vi "Interface Browser.vi"(5 "Caller VI Refnum (Callee's Caller)":refnum<vi>, 7 "Name(\"\" to use uuid)":string="interface_browser") -> ()   [LabVIEW 2017]
uses:
  _Support/Priority Queue/Priority Queue.lvclass/Priority Queue.ctl
  <vilib>/Utility/miscctls.llb/LVPointTypeDef.ctl
  AdvanceAPI/CSM - Check If Module Exists.vi
  Utility/Build Error Cluster.vi
  AdvanceAPI/CSM - Revert Arguments-Safe String.vi
  _Support/Common/Trim Single line Text.vi
  AdvanceAPI/CSM - Make String Arguments Safe.vi
  AdvanceAPI/CSM - Break Down Multiple States String.vi
  AdvanceAPI/CSM - Compact Multiple States.vi
  _Support/CSMQ/_Obtain CSM Data Queue.vi
  _Support/Priority Queue/Release Priority Queue.vi
  AdvanceAPI/CSM - Keywords.vi
  _Support/Priority Queue/Obtain Priority Queue.vi
  _csmHelper/API/Create From VI Reference.vi
  _csmHelper/API/Open Front Panel.vi
  _csmHelper/API/Destroy.vi
  _Support/Error/CSM No Target Error.vi
  _Polymophic/CSM - Filter Duplicated Lines.vi
  _Support/Priority Queue/Priority Queue.lvclass
  Communicable State Machine.lvlib
  _csmHelper/API with lvcsm Support/CSM-Helper API with lvcsm Support.lvlib
  _csmHelper/CSM-Helper.lvclass
  _csmHelper/lvcsmFile/lvcsm File Support.lvlib
panel:
  in  "Opton:All-CSM-VIs":bool
  in  "Scan Project":bool
  in  "Refresh":bool
  in  "Fast Forward":bool
  in  "Fast Reverse":bool
  in  "Skip to Beginning":bool
  in  "Skip to End":bool
  in  "Stop":bool
  in  "Play":bool
  in  "Open":bool
  in  "MainTree":string[](tree)
  in  "Interface-Filter":enum16{"API-Only", "UserDef States", "All"}(ring)=enum."UserDef States"
  in  "CSM-States":i32[](listbox)
  out "StateInfo@Image":string
  out "2D Picture":picture
  out "String":string
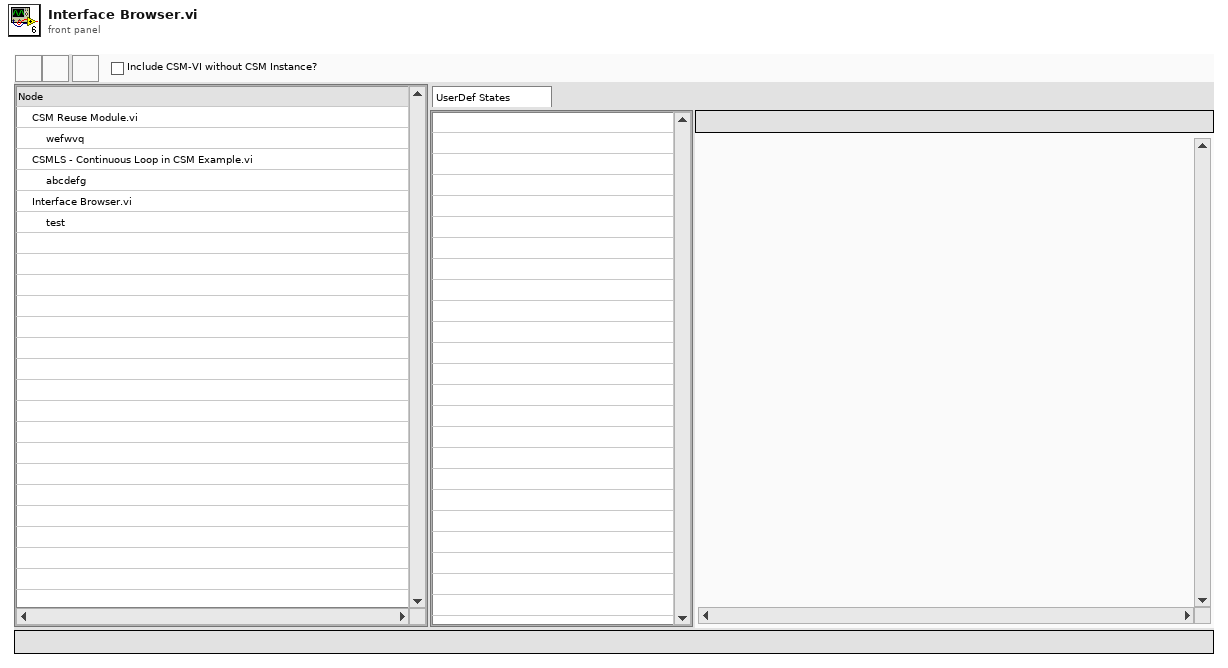
[diagram p1: front panel]
types:
  T1 = enum32{"Invalid", "Standard", "Closed", "Hidden", "Minimized", "Maximized"}
  T2 = enum32{"invalid app kind", "Development System", "Run Time System", "Student Edition", "Embedded LabVIEW", "Evaluation", "Custom"}
  T3 = typedef "LVPointTypeDef.ctl" = cluster{"Horizontal":i16, "Vertical":i16}
  T4 = typedef "Communicable State Machine.lvlib/_CSM_Response Source Message.ctl" = cluster{"‘State":string, "’Arguments":string, "’Error":errorcluster}
  T5 = cluster{"Current VI Reference":refnum<vi>, "Close Panel on Exit?":bool}
  T6 = cluster{"Core":cluster{"Current VI Reference":refnum<vi>, "Close Panel on Exit?":bool}, "Your Boolean data":bool, "Your string data":string}
  T7 = typedef "LVPoint32TypeDef.ctl" = cluster{"Horizontal":i32, "Vertical":i32}
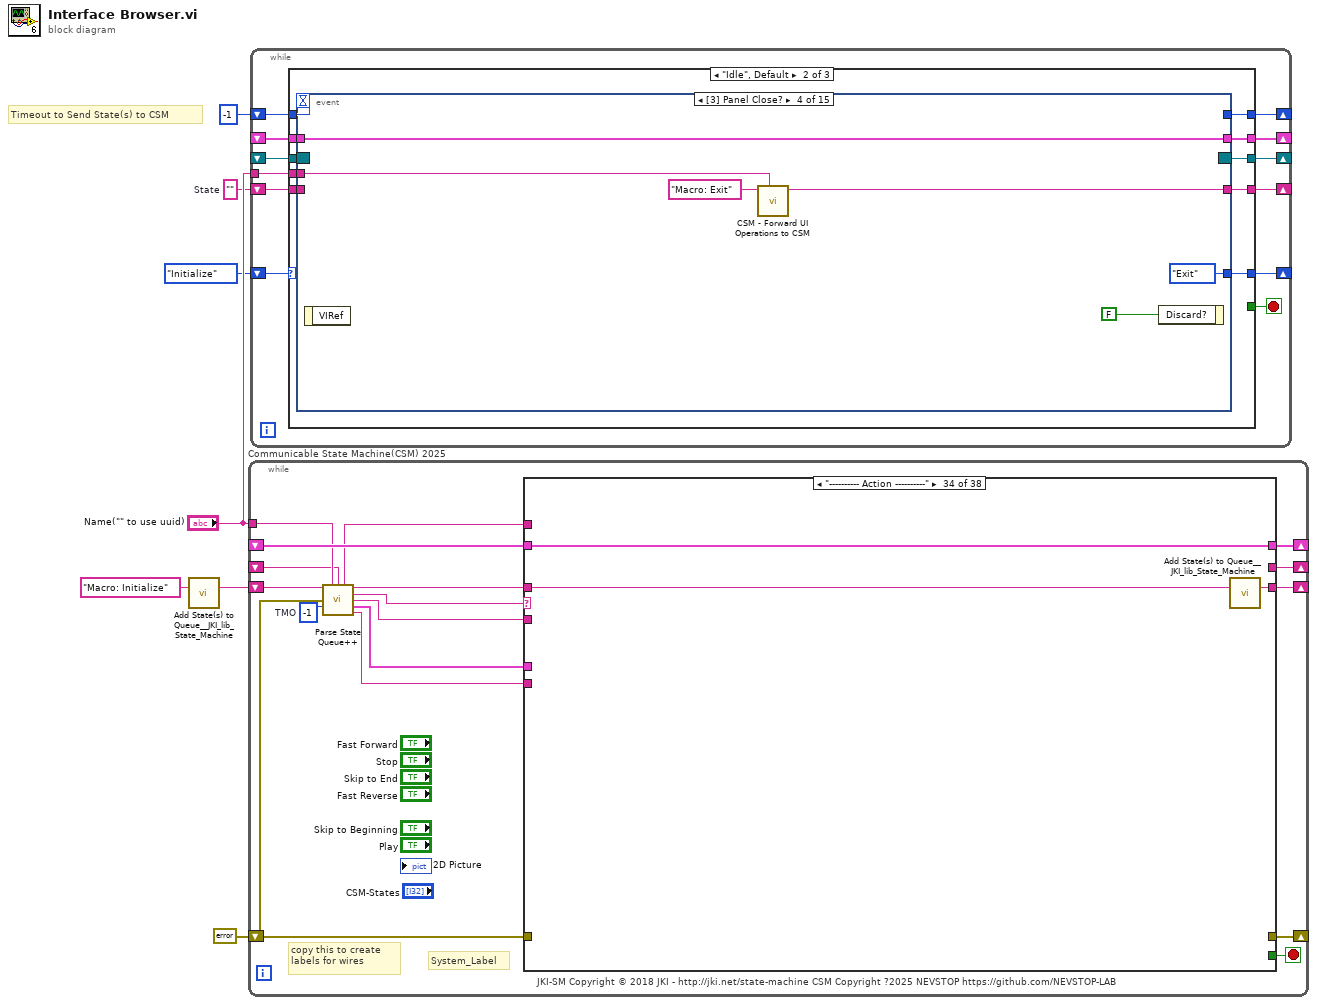
[diagram p0: block diagram]
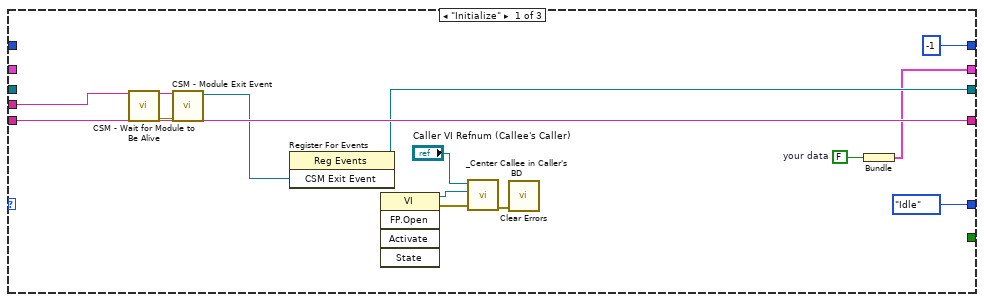
[diagram p2: hidden frame]
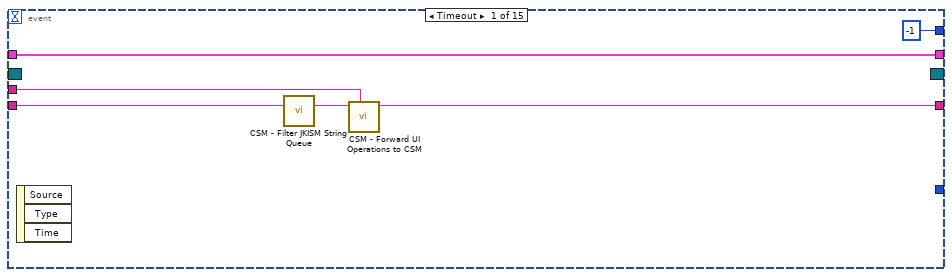
[diagram p3: hidden frame]
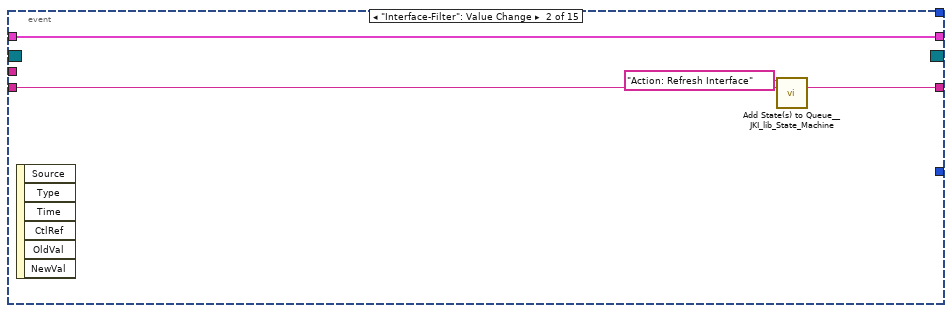
[diagram p4: hidden frame]
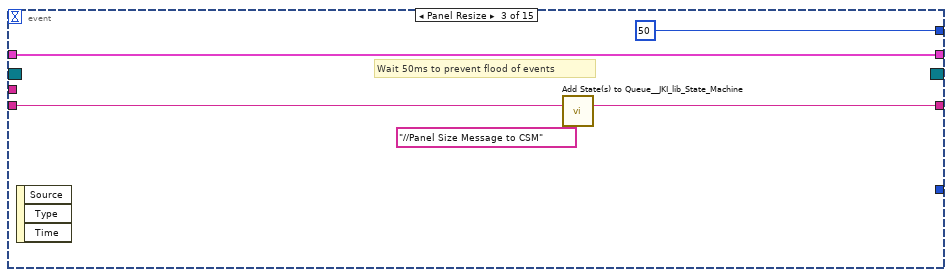
[diagram p5: hidden frame]
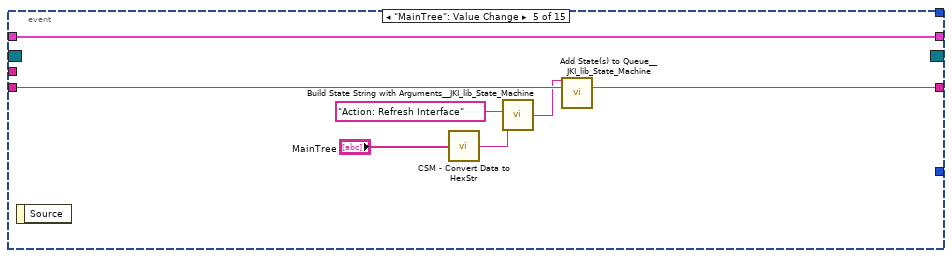
[diagram p6: hidden frame]
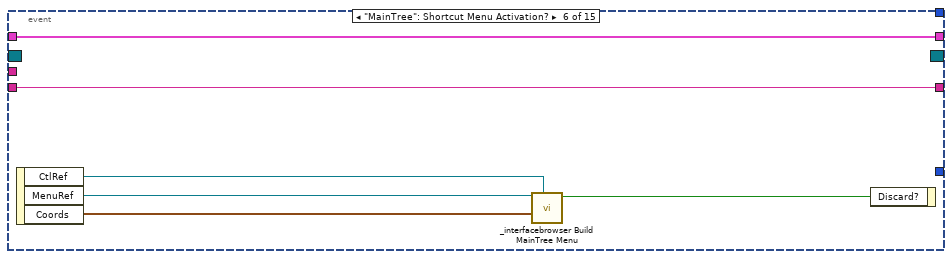
[diagram p7: hidden frame]
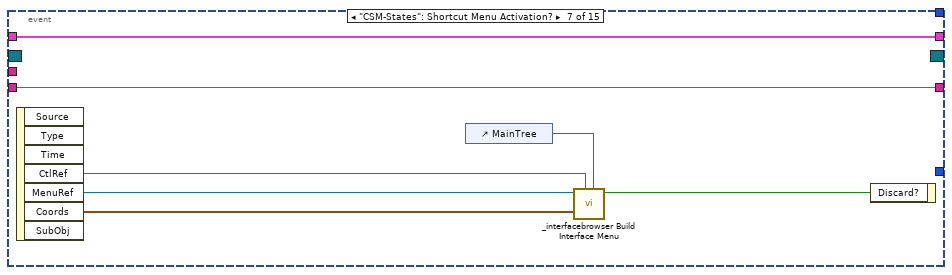
[diagram p8: hidden frame]
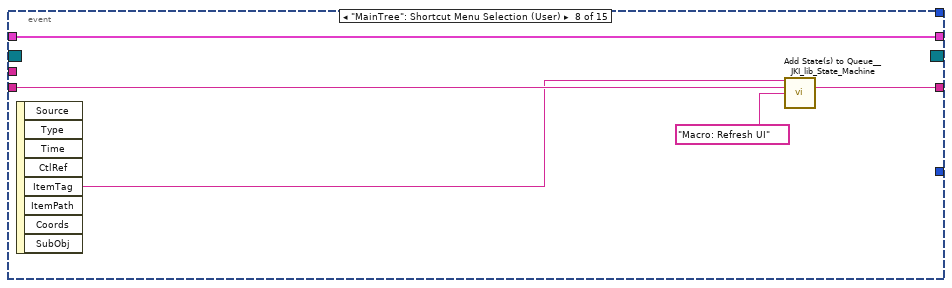
[diagram p9: hidden frame]
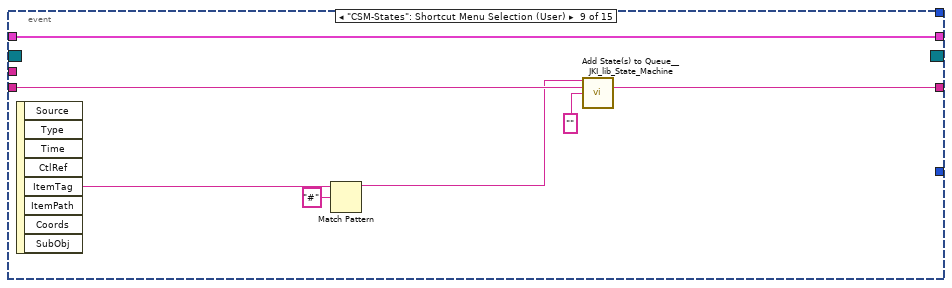
[diagram p10: hidden frame]
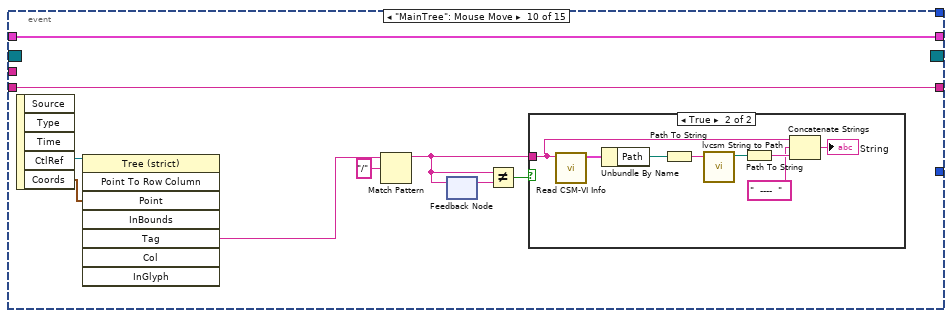
[diagram p11: hidden frame]
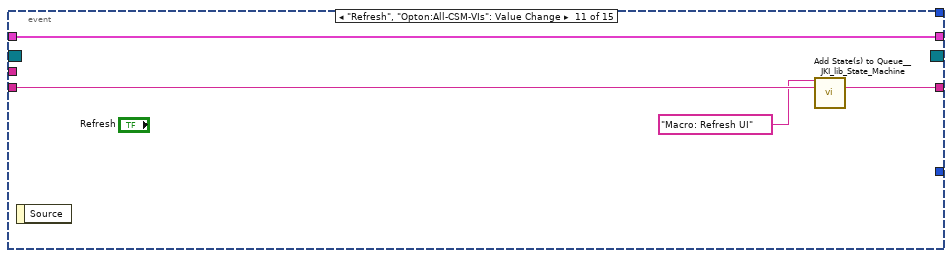
[diagram p13: hidden frame]
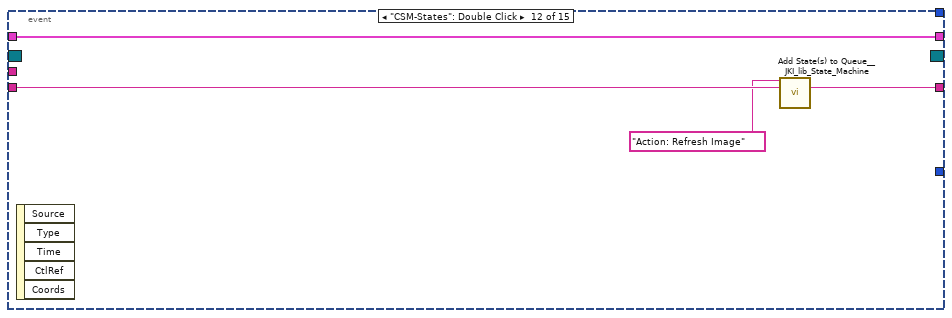
[diagram p14: hidden frame]
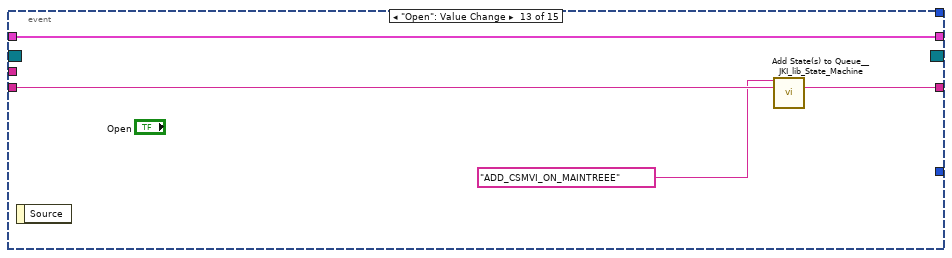
[diagram p15: hidden frame]
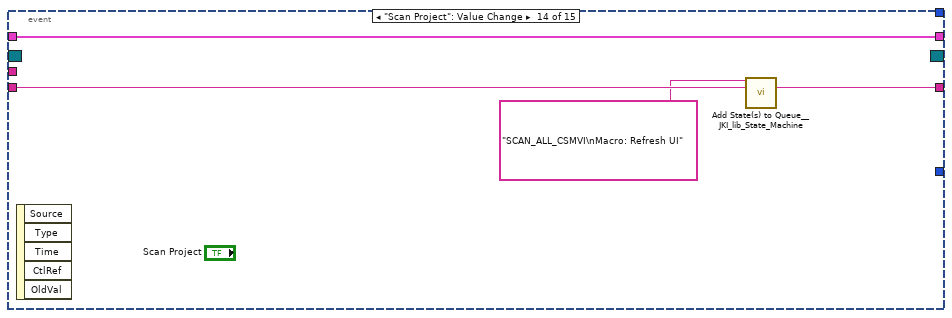
[diagram p16: hidden frame]
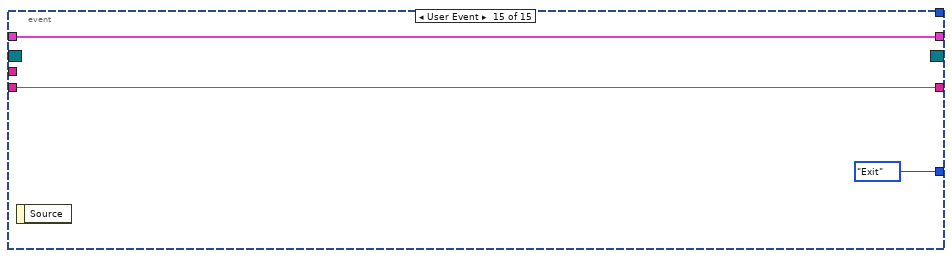
[diagram p17: hidden frame]
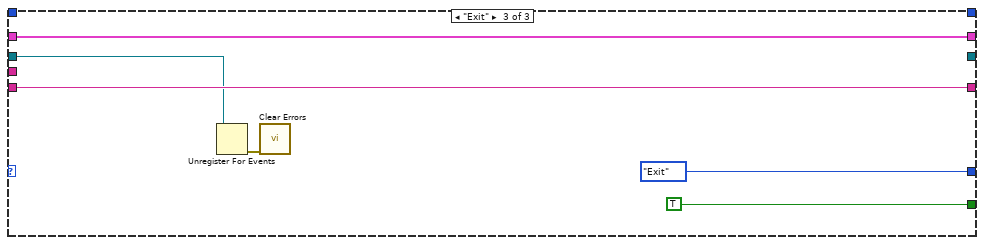
[diagram p18: hidden frame]
diagram:
  w5 = ""  # State
  # "Timeout to Send State(s) to CSM"
  n1 = call <vilib>:"Add State(s) to Queue__JKI_lib_State_Machine.vi"("State(s) in (\"\")"="Macro: Initialize" ("Init State(\"Macro: Initialize\")")) -> ("States Out"=w1:string)  [unwired: 14 in]
  n2 = while "Communicable State Machine(CSM) 2025" {
    shift-right: [w19] -> _
    shift-left: _ -> [w18]
    shift-right: [w22] -> _
    shift-left: errorcluster {"status"=FALSE, "code"=0, "source"=""} ("error out") -> [w8]
    shift-right: [w21] -> _
    shift-left: w1 -> [w23]
    tunnel: "Name(\"\" to use uuid)" -> [w15]
    shift-right: [w16] -> _
    shift-left: _ -> [w10]
    stop <- w20 stop-if-true
    w17 = -1  # TMO
    # "JKI-SM Copyright © 2018 JKI - http://jki.net/state-machine CSM Copyright ?2025 NEVSTOP https://github.com/NEVSTOP-LAB"
    # "copy this to create labels for wires"
    # "System_Label"
    n3 = call "Parse State Queue++.vi"("State Queue"=w23, "Name(\"\" to use uuid)"=w15, "Response Arguments"=w10, "Previous Error"=w8, "Dequeue Timeout(0ms)"=w17) -> ("Name Used"=w9:string, "Remaining States"=w24:string, "Current State"=w11:string, "Arguments"=w12:string, ">> Response Source Message >>"=w13:T4, ">> Source CSM >>"=w14:string)  [unwired: 5 in]
    n4 = case shown="\"---------- Action ----------\"" w11 {
      selector: w11 -> [_ _ _ w35 _ _ _ _ _ _ _ _ _ _ _ _ _ _ _ _ _ _ _ _ _ _ _ _ _ _ _ _ _ _ _ _ _ _]
      tunnel: w24 -> [w25 w28 w31 w39 w44 w50 w73 w79 w85 w95 w102 w114 w118 w121 w127 w131 w137 w140 w144 w148 w154 w156 w166 w180 w187 w204 w216 w237 w251 w258 w278 w280 w283 w286 w297 w308 w321 w352]
      tunnel: w12 -> [_ _ _ _ _ w49 w69 w76 w82 w89 _ _ _ _ _ _ _ _ _ _ _ _ _ _ _ _ _ _ _ _ _ _ _ _ _ _ _ _]
      tunnel: w18 -> [w26 w27 w29 w37 w43 w55 w71 w77 w83 w93 w101 w108 w116 w119 _ w130 w132 w138 w142 w146 w152 w155 w165 w179 w190 w203 w215 w236 w250 w257 w277 w279 w282 w284 w295 w306 w319 w351]
      tunnel: [_ _ _ w32 w45 errorcluster {"status"=FALSE, "code"=0, "source"=""} ("error out") w66 w74 w80 w96 _ _ _ _ _ _ w133 _ _ _ _ w157 w160 w175 _ w195 w208 w222 w244 w256 w276 _ _ _ w287 _ _ w342] -> w22
      tunnel: w8 -> [_ _ _ w33 w45 w53 w67 w75 w81 _ _ _ _ _ _ _ w134 _ _ _ _ w157 _ _ _ _ _ _ _ _ _ _ _ _ _ _ _ _]
      tunnel: [w25 w28 w30 w38 w44 w51 w72 w78 w84 w94 w102 w113 w117 w120 w126 w131 w136 w139 w143 w147 w153 w156 w166 w180 w188 w204 w216 w237 w251 w258 w278 w280 w283 w285 w296 w307 w320 w352] -> w21
      tunnel: [_ _ _ _ _ _ TRUE _ _ _ _ _ TRUE _ _ _ _ _ _ _ _ _ _ _ _ _ _ _ _ _ _ _ _ _ _ _ _ _] -> w20
      tunnel: [w26 w27 w29 w37 w43 w55 w71 w77 w83 w92 w101 w112 w116 w119 w125 w130 w132 w138 w142 w146 w152 w155 w165 w179 w190 w203 w215 w236 w250 w257 w277 w279 w282 w284 w295 w306 w319 w351] -> w19
      tunnel: w14 -> [_ _ _ _ _ w48 _ _ _ w90 _ _ _ _ _ _ _ _ _ _ _ _ _ _ _ _ _ _ _ w253 _ _ _ _ _ _ _ _]
      tunnel: w13 -> [_ _ _ _ _ w47 _ _ _ w91 _ _ _ _ _ _ _ _ _ _ _ _ _ _ _ _ _ _ _ _ _ _ _ _ _ _ _ _]
      tunnel: [_ _ _ "" w40 _ _ _ _ _ _ _ _ _ _ _ _ _ _ _ _ _ _ _ _ _ _ _ _ _ _ _ "API1 Response" _ _ _ _ _] -> w16
      tunnel: w9 -> [_ _ _ w34 _ _ w68 _ _ _ _ _ _ _ _ _ _ _ _ _ _ _ _ _ _ _ _ _ _ _ _ _ _ _ _ _ _ _]
      frame "", "Idle" {
      }
      frame "CSM Documentation" {
      }
      frame "---------- Core ----------" {
        n5 = call <vilib>:"Add State(s) to Queue__JKI_lib_State_Machine.vi"("State(s) in (\"\")"=w31) -> ("States Out"=w30:string)  [unwired: 14 in]
      }
      frame Default {
        n6 = call "CSM Unhandled State Error.vi"("error in (no error)"=w33, "Current State"=w35, "CSM Name"=w34) -> ("error out"=w32:errorcluster)  [unwired: 8 in]
        n7 = call <vilib>:"Add State(s) to Queue__JKI_lib_State_Machine.vi"("State(s) in (\"\")"=w39) -> ("States Out"=w38:string)  [unwired: 14 in]
      }
      frame "VI Reference" {
        n8 = Unbundle By Name(w43) -> ("Core"=w42:T5)
        n9 = Unbundle By Name(w42) -> ("Current VI Reference"=w41:refnum<vi>)
        n10 = call "CSM - Convert Data to HexStr.vi"("Variant"=w41) -> ("HEX String (0-9,A-F)"=w40:string)  [unwired: 8 in]
      }
      frame "Error Handler" {
        # "Clear error"
        n11 = case shown="Error" w53 {
          selector: w53 -> [_ w60]
          tunnel: [w59 w62] -> w52
          tunnel: w50 -> [w59 w61]
          tunnel: w49 -> [w58 _]
          tunnel: w48 -> [_ _]
          tunnel: w47 -> [_ _]
          tunnel: [w57 w60] -> w46
          frame No Error {
            n12 = call "CSM - Convert Argument to Error.vi"("Argument"=w58) -> ("error"=w57:errorcluster)  [unwired: 4 in]
            n13 = flat-sequence {
              tunnel: w57 -> [_]
              frame #0 {
              }
            }
          }
          frame Error {
            n14 = call "CSM - Convert Error to Argument.vi"("error"=w60) -> ("Argument"=w64:string)  [unwired: 4 in]
            n15 = call <vilib>:"Build State String with Arguments__JKI_lib_State_Machine.vi"("Arguments (\"\")"=w64, "State"="Error Occurred" ("Status with Arguments")) -> ("State with Arguments"=w63:string)  [unwired: 4 in]
            n16 = call "CSM - Broadcast Status Change.vi"("Status with Arguments"=w63, "State Queue"=w61) -> ("Remaining States"=w62:string)  [unwired: 13 in]
          }
        }
        n17 = call <vilib>:"Simple Error Handler.vi"("error in (no error)"=w46) -> ()  [unwired: 4 in, 5 out]
        n18 = call <vilib>:"Add State(s) to Queue__JKI_lib_State_Machine.vi"("State(s) in Front (\"\")"="// Post Error States", "State(s) in (\"\")"=w52) -> ("States Out"=w51:string)  [unwired: 13 in]
      }
      frame "Critical Error" {
        n19 = call "CSM Critical Error.vi"("error in (no error)"=w67, "Arugments(as Reason)"=w69, "CSM Name"=w68) -> ("error out"=w66:errorcluster)  [unwired: 8 in]
        n20 = call <vilib>:"Add State(s) to Queue__JKI_lib_State_Machine.vi"("State(s) in (\"\")"=w73) -> ("States Out"=w72:string)  [unwired: 14 in]
      }
      frame "Target Timeout Error" {
        n21 = call "CSM Target Timeout Error.vi"("error in (no error)"=w75, "Arguments(as CSM Name)"=w76) -> ("error out"=w74:errorcluster)  [unwired: 9 in]
        n22 = call <vilib>:"Add State(s) to Queue__JKI_lib_State_Machine.vi"("State(s) in (\"\")"=w79) -> ("States Out"=w78:string)  [unwired: 14 in]
      }
      frame "Target Error" {
        n23 = call "CSM Target Error.vi"("error in (no error)"=w81, "Arguments(as CSM Name)"=w82) -> ("error out"=w80:errorcluster)  [unwired: 9 in]
        n24 = call <vilib>:"Add State(s) to Queue__JKI_lib_State_Machine.vi"("State(s) in (\"\")"=w85) -> ("States Out"=w84:string)  [unwired: 14 in]
      }
      frame "Async Response", "Response" {
        n25 = Unbundle(w91) -> ("‘State"=w88:string, "’Arguments"=w87:string, "’Error"=w86:errorcluster)
        n26 = case shown="Default" w88 {
          tunnel: [w97] -> w94
          tunnel: w95 -> [w98]
          tunnel: [w100] -> w92
          tunnel: w93 -> [w100]
          tunnel: [w99] -> w96
          tunnel: w86 -> [w99]
          tunnel: w90 -> [_]
          tunnel: w89 -> [_]
          tunnel: w87 -> [_]
          frame Default {
            n27 = call <vilib>:"Add State(s) to Queue__JKI_lib_State_Machine.vi"("State(s) in (\"\")"=w98) -> ("States Out"=w97:string)  [unwired: 14 in]
          }
        }
      }
      frame "Async Message Posted" {
      }
      frame "Initialize Core Data" {
        # "originally closed?"
        # "exe?"
        # "If panel starts closed or is an EXE, then close it when we exit"
        n28 = control-ref of="Current VI Reference"() -> (w106:refnum<vi>)
        n29 = property class="VI"() -> ("FP.State"=w105:T1)  [unwired: 2 in, 2 out]
        n30 = property class="App"() -> ("App.Kind"=w111:T2)  [unwired: 2 in, 2 out]
        n31 = Equal?(x=w105, y=T1."Closed" ("Front Panel Window:State")) -> (x = y?=w103:bool)
        n32 = Equal?(x=w111, y=T2."Run Time System" ("Application:Kind")) -> (x = y?=w109:bool)
        n33 = Or(x=w103, y=w109) -> (x .or. y?=w107:bool)
        n34 = Bundle By Name(cluster=w108, "Core.Current VI Reference"=w106, "Core.Close Panel on Exit?"=w107) -> (w112:T6)
        n35 = call <vilib>:"Add State(s) to Queue__JKI_lib_State_Machine.vi"("State(s) in (\"\")"=w114) -> ("States Out"=w113:string)  [unwired: 14 in]
      }
      frame "Exit" {
        n36 = call <vilib>:"Add State(s) to Queue__JKI_lib_State_Machine.vi"("State(s) in (\"\")"=w118) -> ("States Out"=w117:string)  [unwired: 14 in]
      }
      frame "---------- Data ----------" {
        n37 = call <vilib>:"Add State(s) to Queue__JKI_lib_State_Machine.vi"("State(s) in (\"\")"=w121) -> ("States Out"=w120:string)  [unwired: 14 in]
      }
      frame "Data: Initialize" {
        w122 = T5 {"Current VI Reference"=refnum, "Close Panel on Exit?"=FALSE}  # Core
        w124 = TRUE  # Your Boolean data
        w123 = ""  # Your string data
        n38 = Bundle("Core"=w122, "Your Boolean data"=w124, "Your string data"=w123) -> (w125:T6)  [unwired: 1 in]
        n39 = call <vilib>:"Add State(s) to Queue__JKI_lib_State_Machine.vi"("State(s) in (\"\")"=w127) -> ("States Out"=w126:string)  [unwired: 14 in]
      }
      frame "Data: Update Indicators" {
        n40 = local write "2D Picture"(picture data[5B] ("2D Picture 2")) -> ()
        n41 = property on="2D Picture" class="Pict"("Origin"=T3 {"Horizontal"=0, "Vertical"=0}) -> ()  [unwired: 2 in, 2 out]
      }
      frame "Data: Cleanup" {
        n42 = Unbundle By Name(w132) -> ("Core.Current VI Reference"=w135:refnum<vi>)
        n43 = Close Reference(reference=w135, error in (no error)=w134) -> (error out=w133:errorcluster)
        n44 = call <vilib>:"Add State(s) to Queue__JKI_lib_State_Machine.vi"("State(s) in (\"\")"=w137) -> ("States Out"=w136:string)  [unwired: 14 in]
      }
      frame "---------- Macro ----------" {
        n45 = call <vilib>:"Add State(s) to Queue__JKI_lib_State_Machine.vi"("State(s) in (\"\")"=w140) -> ("States Out"=w139:string)  [unwired: 14 in]
      }
      frame "Macro: Initialize" {
        n46 = call <vilib>:"Add State(s) to Queue__JKI_lib_State_Machine.vi"("State(s) in Front (\"\")"="Data: Initialize\nInitialize Core Data\nData: Update Indicators\nMacro: Refresh UI", "State(s) in (\"\")"=w144) -> ("States Out"=w143:string)  [unwired: 13 in]
      }
      frame "Macro: Refresh UI" {
        n47 = call <vilib>:"Add State(s) to Queue__JKI_lib_State_Machine.vi"("State(s) in Front (\"\")"="Action: Refresh(CSM-VI mode)\nAction: Refresh Interface\nAction: Refresh Image", "State(s) in (\"\")"=w148) -> ("States Out"=w147:string)  [unwired: 13 in]
      }
      frame "Macro: Exit" {
        n48 = call <vilib>:"Add State(s) to Queue__JKI_lib_State_Machine.vi"("State(s) in Front (\"\")"="//Exit Sub-Modules ", "State(s) at Back (\"\")"="Data: Cleanup\nExit") -> ("States Out"=w150:string)  [unwired: 13 in]
        n49 = call <vilib>:"Add State(s) to Queue__JKI_lib_State_Machine.vi"("State(s) in Front (\"\")"=w150, "State(s) in (\"\")"=w154) -> ("States Out"=w153:string)  [unwired: 13 in]
      }
      frame "------ Menu Handler ------" {
      }
      frame "ADD_CSM_ON_CSMVI" {
        n50 = control-ref of="MainTree"() -> (w164:refnum<vi>)
        n51 = property class="Tree (strict)"(reference=w164) -> ("Value"=w163:string[])  [unwired: 1 in, 2 out]
        n52 = call "CSM Module Name"() -> ("CSM Module"=w161:string, "OK"=w159:bool)  [unwired: 17 in, 1 out]
        n53 = Index Array(array=w163) -> (element=w162:string)  [unwired: 1 in]
        n54 = call <vilib>:"Trim Whitespace.vi"("string"=w161) -> ("trimmed string"=w158:string)  [unwired: 1 in]
        n55 = case shown="True" w159 {
          tunnel: w162 -> [_ w169]
          tunnel: w158 -> [_ w168]
          tunnel: [_ w167] -> w160
          frame False {
          }
          frame True {
            n56 = call "Add CSM Module.vi"("CSM-VI"=w169, "CSM Name"=w168) -> ("error out"=w167:errorcluster)  [unwired: 9 in]
          }
        }
      }
      frame "ADD_CSM_ON_CSM" {
        n57 = control-ref of="MainTree"() -> (w178:refnum<vi>)
        n58 = property class="Tree (strict)"(reference=w178) -> ("Value"=w177:string[])  [unwired: 1 in, 2 out]
        n59 = Index Array(array=w177) -> (element=w172:string)  [unwired: 1 in]
        n60 = call "CSM Module Name2"() -> ("CSM Module"=w176:string, "OK"=w174:bool)  [unwired: 17 in, 1 out]
        n61 = Match Pattern(string=w172, regular expression="/") -> (before substring=w171:string)  [unwired: 1 in, 3 out]
        n62 = call <vilib>:"Trim Whitespace.vi"("string"=w176) -> ("trimmed string"=w173:string)  [unwired: 1 in]
        n63 = case shown="True" w174 {
          tunnel: w171 -> [_ w183]
          tunnel: w173 -> [_ w182]
          tunnel: [_ w181] -> w175
          frame False {
          }
          frame True {
            n64 = call "Add CSM Module.vi"("CSM-VI"=w183, "CSM Name"=w182) -> ("error out"=w181:errorcluster)  [unwired: 9 in]
          }
        }
      }
      frame "ADD_CSMVI_ON_MAINTREEE" {
        n65 = call "File Dialog"("pattern (all files)"="*.vi") -> ("selected path"=w185:path, "error out"=w186:errorcluster)  [unwired: 11 in, 2 out]
        n66 = case shown="Error" w186 {
          selector: w186 -> [w193 _]
          tunnel: w185 -> [w194 _]
          tunnel: ["Macro: Refresh UI" ("State(s) in Front (\"\")") _] -> w184
          frame No Error {
            n67 = call "Add CSM-VI.vi"("error in (no error)"=w193, "CSM-VI"=w194) -> ("error out"=w191:errorcluster)  [unwired: 9 in]
            n68 = call <vilib>:"Simple Error Handler.vi"("error in (no error)"=w191) -> ()  [unwired: 4 in, 5 out]
          }
          frame Error {
          }
        }
        n69 = call <vilib>:"Add State(s) to Queue__JKI_lib_State_Machine.vi"("State(s) in Front (\"\")"=w184, "State(s) in (\"\")"=w187) -> ("States Out"=w188:string)  [unwired: 13 in]
      }
      frame "RM_CSM_ON_CSM" {
        n70 = control-ref of="MainTree"() -> (w202:refnum<vi>)
        n71 = property class="Tree (strict)"(reference=w202) -> ("Value"=w201:string[])  [unwired: 1 in, 2 out]
        n72 = Index Array(array=w201) -> (element=w200:string)  [unwired: 1 in]
        n73 = Two Button Dialog(message="Are you sure to remove it?") -> (T button?=w196:bool)  [unwired: 2 in]
        n74 = Match Pattern(string=w200, regular expression="/") -> (after substring=w197:string)  [unwired: 1 in, 3 out]
        n75 = case shown="True" w196 {
          tunnel: w197 -> [_ w206]
          tunnel: [_ w205] -> w195
          frame False {
          }
          frame True {
            n76 = call "Delete CSM Module.vi"("CSM Name"=w206) -> ("error out"=w205:errorcluster)  [unwired: 10 in]
          }
        }
      }
      frame "RM_CSMVI_ON_CSMVI" {
        n77 = control-ref of="MainTree"() -> (w214:refnum<vi>)
        n78 = property class="Tree (strict)"(reference=w214) -> ("Value"=w213:string[])  [unwired: 1 in, 2 out]
        n79 = Index Array(array=w213) -> (element=w212:string)  [unwired: 1 in]
        n80 = Two Button Dialog(message="Are you sure to remove it?") -> (T button?=w209:bool)  [unwired: 2 in]
        n81 = Match Pattern(string=w212, regular expression="/") -> (before substring=w207:string)  [unwired: 1 in, 3 out]
        n82 = case shown="True" w209 {
          tunnel: w207 -> [_ w218]
          tunnel: [_ w217] -> w208
          frame False {
          }
          frame True {
            n83 = call "Delete CSM-VI.vi"("CSM Name"=w218) -> ("error out"=w217:errorcluster)  [unwired: 10 in]
          }
        }
      }
      frame "OPEN_CSMVI_ON_CSM", "OPEN_CSMVI_ON_CSMVI" {
        n84 = control-ref of="MainTree"() -> (w235:refnum<vi>)
        n85 = property class="Tree (strict)"(reference=w235) -> ("Value"=w234:string[])  [unwired: 1 in, 2 out]
        n86 = Index Array(array=w234) -> (element=w233:string)  [unwired: 1 in]
        n87 = Match Pattern(string=w233, regular expression="/") -> (before substring=w231:string)  [unwired: 1 in, 3 out]
        n88 = call "Read CSM-VI Info.vi"("CSM Name"=w231) -> ("Cluster 2"=w230:cluster{"Path":path})  [unwired: 9 in, 1 out]
        n89 = Unbundle By Name(w230) -> ("Path"=w220:path)
        n90 = Path To String(path=w220) -> (string=w219:string)
        n91 = call "lvcsm String to Path.vi"("common path"=w219) -> ("Path"=w221:path)  [unwired: 10 in]
        n92 = Open VI Reference(vi path=w221, options=2) -> (vi reference=w228:refnum<vi>, error out=w227:errorcluster)  [unwired: 4 in]
        n93 = call-poly "CSM-Helper API.vi"("error in (no error)"=w227, "VI"=w228) -> ("error out"=w225:errorcluster, "CSM-Helper.lvclass"=w226:refnum<class "CSM-Helper.lvclass">)  [unwired: 8 in]
        n94 = call-poly "CSM-Helper API.vi"("error in (no error)"=w225, "CSM-Helper in"=w226) -> ("error out"=w223:errorcluster, "CSM-Helper out"=w224:refnum<class "CSM-Helper.lvclass">)  [unwired: 8 in]
        n95 = call-poly "CSM-Helper API.vi"("error in (no error)"=w223, "CSM-Helper in"=w224) -> ("error out"=w222:errorcluster)  [unwired: 8 in, 1 out]
      }
      frame "GOTO_ON_CSMSTATE" {
        n96 = control-ref of="MainTree"() -> (w243:refnum<vi>)
        n97 = control-ref of="CSM-States"() -> (w248:refnum<vi>)
        n98 = property class="LstBox (strict)"(reference=w248) -> ("Item Names"=w249:string[], "Value"=w247:i32[])  [unwired: 1 in, 2 out]
        n99 = property class="Tree (strict)"(reference=w243) -> ("Value"=w242:string[])  [unwired: 1 in, 2 out]
        n100 = Index Array(array=w247) -> (element=w246:i32)  [unwired: 1 in]
        n101 = Index Array(array=w242) -> (element=w241:string)  [unwired: 1 in]
        n102 = Index Array(array=w249, index=w246) -> (element=w245:string)
        n103 = Match Pattern(string=w241, regular expression="/") -> (before substring=w239:string)  [unwired: 1 in, 3 out]
        n104 = call "Jump to CSM State.vi"("Type"=enum16{"CSM", "CSM-VI"}."CSM-VI", "State"=w245, "Name"=w239) -> ("Error out"=w244:errorcluster)  [unwired: 8 in]
      }
      frame "SCAN_ALL_CSMVI" {
        n105 = case shown="\"\"" w253 {
          selector: w253 -> [w260 _]
          tunnel: [w259 w261] -> w252
          frame Default {
            n106 = call "lvcsm String to Path.vi"("common path"=w260) -> ("Path"=w259:path)  [unwired: 10 in]
          }
          frame "" {
            n107 = property class="App"() -> ("Project.ActiveProject"=w263:refnum<vi>)  [unwired: 2 in, 2 out]
            n108 = property class="Project"(reference=w263) -> ("Path"=w262:path)  [unwired: 1 in, 2 out]
            n109 = Strip Path(path=w262) -> (stripped path=w261:path)  [unwired: 1 out]
          }
        }
        n110 = Two Button Dialog(message="Scan for CSM Modules?") -> (T button?=w254:bool)  [unwired: 2 in]
        n111 = case shown="True" w254 {
          tunnel: [_ w265] -> w256
          tunnel: w252 -> [_ w264]
          frame False {
          }
          frame True {
            n112 = call "Scan CSM-VI.vi"("root"=w264) -> ("Error out"=w265:errorcluster)  [unwired: 10 in]
          }
        }
      }
      frame "RESCAN_INTERFACE_ON_CSMVI" {
        n113 = control-ref of="MainTree"() -> (w275:refnum<vi>)
        n114 = property class="Tree (strict)"(reference=w275) -> ("Value"=w274:string[])  [unwired: 1 in, 2 out]
        n115 = Index Array(array=w274) -> (element=w273:string)  [unwired: 1 in]
        n116 = Match Pattern(string=w273, regular expression="/") -> (before substring=w271:string)  [unwired: 1 in, 3 out]
        n117 = call "Read CSM-VI Info.vi"("CSM Name"=w271) -> ("error out"=w266:errorcluster, "Cluster 2"=w270:cluster{"Path":path})  [unwired: 9 in]
        n118 = Unbundle By Name(w270) -> ("Path"=w268:path)
        n119 = Path To String(path=w268) -> (string=w269:string)
        n120 = call "lvcsm String to Path.vi"("common path"=w269) -> ("Path"=w267:path)  [unwired: 10 in]
        n121 = call "Add CSM-VI.vi"("error in (no error)"=w266, "CSM-VI"=w267) -> ("error out"=w276:errorcluster)  [unwired: 9 in]
      }
      frame "---------- API ----------" {
      }
      frame "API: API1" {
      }
      frame "---------- Action ----------" {
        n122 = call <vilib>:"Add State(s) to Queue__JKI_lib_State_Machine.vi"("State(s) in (\"\")"=w286) -> ("States Out"=w285:string)  [unwired: 14 in]
      }
      frame "Action: Refresh(CSM mode)" {
        n123 = control-ref of="MainTree"() -> (w294:refnum<vi>)
        n124 = call "_interfacebrowser build tree table in CSM mode.vi"() -> ("Error out"=w287:errorcluster, "Type"=w288:string[], "Tree Table"=w289:string[][])  [unwired: 9 in]
        n125 = call "MGI Populate Tree with Delimited Strings_csm.vi"("Default Symbol"=17, "Delimiter"="/", "Items (Delimited)"=w289, "Tree Control"=w294) -> ("error out"=w291:errorcluster, "Tree Control Dup"=w290:refnum<vi>)  [unwired: 5 in, 1 out]
        n126 = property class="Tree"(reference=w290, error in=w291, "RowHdrs[]"=w288) -> ()  [unwired: 2 out]
        n127 = call <vilib>:"Add State(s) to Queue__JKI_lib_State_Machine.vi"("State(s) in (\"\")"=w297) -> ("States Out"=w296:string)  [unwired: 14 in]
      }
      frame "Action: Refresh(CSM-VI mode)" {
        n128 = call "_interfacebrowser build tree table in CSM-VI mode.vi"("Opton:All-CSM-VIs"="Opton:All-CSM-VIs") -> ("Type"=w299:string[], "Tree Table"=w300:string[][])  [unwired: 8 in, 1 out]
        n129 = control-ref of="MainTree"() -> (w305:refnum<vi>)
        n130 = call "MGI Populate Tree with Delimited Strings_csm.vi"("Default Symbol"=17, "Delimiter"="/", "Items (Delimited)"=w300, "Tree Control"=w305) -> ("error out"=w302:errorcluster, "Tree Control Dup"=w301:refnum<vi>)  [unwired: 5 in, 1 out]
        n131 = property class="Tree"(reference=w301, error in=w302, "RowHdrs[]"=w299) -> ()  [unwired: 2 out]
        n132 = call <vilib>:"Add State(s) to Queue__JKI_lib_State_Machine.vi"("State(s) in (\"\")"=w308) -> ("States Out"=w307:string)  [unwired: 14 in]
      }
      frame "Action: Refresh Interface" {
        n133 = control-ref of="MainTree"() -> (w310:refnum<vi>)
        n134 = property class="Tree (strict)"(reference=w310) -> ("Value"=w309:string[])  [unwired: 1 in, 2 out]
        n135 = for {
          tunnel: [w334] -> w318 mode=indexing
          tunnel: w309 -> [w332] mode=indexing
          n136 = Match Pattern(string=w332, regular expression="/") -> (before substring=w331:string)  [unwired: 1 in, 3 out]
          n137 = call "Read CSM States By CSM-VI.vi"("CSM VI"=w331) -> ("Array"=w335:string[])  [unwired: 9 in, 1 out]
          n138 = Bundle("Array"=w335) -> (w334:cluster{"Array":string[]})  [unwired: 1 in]
        }
        n139 = Delete From Array(array=w318, index=0) -> (deleted portion=w315:cluster{"Array":string[]}, array with subset deleted=w316:cluster{"Array":string[]}[])  [unwired: 1 in]
        n140 = Unbundle(w315) -> ("Array"=w314:string[])
        n141 = for {
          tunnel: w316 -> [w327] mode=indexing
          shift-right: [w322] -> w313
          shift-left: w314 -> [w326]
          n142 = Unbundle(w327) -> ("Array"=w325:string[])
          n143 = Build Array (concatenate)(w326, w325) -> (w323:string[])
          n144 = call "Remove Duplicates String Item_csm.vi"("Input Array"=w323) -> ("indices of removed elements"=w324:i32[])  [unwired: 1 out]
          n145 = for {
            tunnel: w324 -> [w329] mode=indexing
            tunnel: w323 -> [w330]
            tunnel: [w328] -> w322 mode=indexing
            n146 = Index Array(array=w330, index=w329) -> (element=w328:string)
          }
        }
        n147 = call "_interfacebrowser filter CSM States.vi"("Interface-Filter"="Interface-Filter", "Array"=w313) -> ("filtered array"=w312:string[])  [unwired: 9 in]
        n148 = property on="CSM-States" class="LstBox (strict)"("Item Names"=w312) -> ()  [unwired: 2 in, 2 out]
        n149 = call <vilib>:"Add State(s) to Queue__JKI_lib_State_Machine.vi"("State(s) in (\"\")"=w321) -> ("States Out"=w320:string)  [unwired: 14 in]
      }
      frame "Action: Refresh Image" {
        n150 = control-ref of="CSM-States"() -> (w349:refnum<vi>)
        n151 = property class="LstBox (strict)"(reference=w349) -> ("Item Names"=w350:string[], "Value"=w348:i32[])  [unwired: 1 in, 2 out]
        n152 = control-ref of="MainTree"() -> (w346:refnum<vi>)
        n153 = property class="Tree (strict)"(reference=w346) -> ("Value"=w345:string[])  [unwired: 1 in, 2 out]
        n154 = Index Array(array=w348) -> (element=w347:i32)  [unwired: 1 in]
        n155 = Index Array(array=w345) -> (element=w344:string)  [unwired: 1 in]
        n156 = Match Pattern(string=w344, regular expression="/") -> (before substring=w340:string)  [unwired: 1 in, 3 out]
        n157 = Index Array(array=w350, index=w347) -> (element=w339:string)
        n158 = Empty String/Path?(string/path=w340) -> (empty?=w338:bool)
        n159 = Empty String/Path?(string/path=w339) -> (empty?=w337:bool)
        n160 = Or(x=w338, y=w337) -> (x .or. y?=w336:bool)
        n161 = case shown="False" w336 {
          tunnel: [w359 _] -> w342
          tunnel: [w358 _] -> w341
          tunnel: w340 -> [w356 _]
          tunnel: w339 -> [w355 _]
          frame False {
            n162 = control-ref of="2D Picture"() -> (w354:refnum<vi>)
            n163 = Format Into String(format string="%s@%s", w355, w356) -> (resulting string=w358:string)  [unwired: 2 in, 1 out]
            n164 = call "Update Case Frame to Image.vi"("Picture Control Reference"=w354, "Type"=enum16{"CSM", "CSM-VI"}."CSM-VI", "State"=w355, "Name"=w356) -> ("Error out"=w359:errorcluster)  [unwired: 7 in]
          }
          frame True {
          }
        }
        "StateInfo@Image" <- w341
      }
    }
  }
  n165 = while {
    shift-right: [w370] -> _
    shift-left: enum16{"Idle", "Initialize", "Exit"}."Initialize" -> [w371]
    tunnel: "Name(\"\" to use uuid)" -> [w368]
    shift-right: [w366] -> _
    shift-left: w5 -> [w367]
    shift-right: [w364] -> _
    shift-left: -1 -> [w365]
    shift-right: [w363] -> _
    shift-left: _ -> [w362]
    shift-right: [w361] -> _
    shift-left: _ -> [w360]
    stop <- w369 stop-if-true
    n166 = case shown="\"Idle\", Default" w371 {
      tunnel: [enum16{"Idle", "Initialize", "Exit"}."Idle" w395 enum16{"Idle", "Initialize", "Exit"}."Exit"] -> w370
      tunnel: [_ _ TRUE] -> w369
      tunnel: w368 -> [w381 w394 _]
      tunnel: w367 -> [w384 w392 w488]
      tunnel: [w384 w393 w488] -> w366
      tunnel: w365 -> [_ w390 _]
      tunnel: [-1 w391 _] -> w364
      tunnel: [w380 w388 _] -> w363
      tunnel: w362 -> [_ w389 w487]
      tunnel: [w376 w386 w485] -> w361
      tunnel: w360 -> [_ w387 w485]
      frame "Initialize" {
        w377 = FALSE  # your data
        n167 = call "CSM - Wait for Module to Be Alive.vi"("CSM Name"=w381) -> ("CSM Name(dup)"=w379:string, "error out"=w378:errorcluster)  [unwired: 12 in, 1 out]
        n168 = call "CSM - Module Exit Event.vi"("Error in"=w378, "Name(\"\" to use uuid) in"=w379) -> ("CSM Exit Event"=w382:refnum<user-event>)  [unwired: 8 in, 1 out]
        n169 = register-events(w382) -> (reference out=w380:refnum<event-registration>)  [unwired: 2 in, 1 out]
        n170 = invoke class="VI" method="FP.Open"() -> (reference out=w373:refnum<vi>, error out=w374:errorcluster)  [unwired: 5 in, 3 out]
        n171 = call "_Center Callee in Caller's BD.vi"("Error In"=w374, "Callee VI Refnum (Caller)"=w373, "Caller VI Refnum (Callee's Caller)"="Caller VI Refnum (Callee's Caller)") -> ("Error Out"=w375:errorcluster)  [unwired: 8 in]
        n172 = call <vilib>:"Clear Errors.vi"("error in (no error)"=w375) -> ()  [unwired: 5 in, 2 out]
        n173 = Bundle("your data"=w377) -> (w376:cluster{"your data":bool})  [unwired: 1 in]
      }
      frame "Idle", Default {
        n174 = event shown="[3] Panel Close?" {
          selector: w389 -> [_ _ _ _ _ _ _ _ _ _ _ _ _ _ _]
          dyn-events: [_ _ _ _ _ _ _ _ _ _ _ _ _ _ _] -> w388
          timeout: w390 -> [_ _ _ _ _ _ _ _ _ _ _ _ _ _ _]
          tunnel: [_ _ _ enum16{"Idle", "Initialize", "Exit"}."Exit" _ _ _ _ _ _ _ _ _ _ enum16{"Idle", "Initialize", "Exit"}."Exit"] -> w395
          tunnel: w394 -> [w397 _ _ w413 _ _ _ _ _ _ _ _ _ _ _]
          tunnel: w392 -> [w400 w403 w410 _ w421 w429 w436 w439 w446 w457 w467 w471 w475 w479 w484]
          tunnel: [w398 w404 w409 w412 w422 w429 w436 w440 w447 w457 w468 w472 w476 w480 w484] -> w393
          tunnel: [-1 _ 50 _ _ _ _ _ _ _ _ _ _ _ _] -> w391
          tunnel: w387 -> [w396 w405 w406 w411 w423 w428 w435 w441 w448 w456 w469 w473 w477 w481 w482]
          tunnel: [w396 w405 w406 w411 w423 w428 w435 w441 w448 w456 w469 w473 w477 w481 w482] -> w386
          event Timeout {
            n175 = event-data() -> ()  [unwired: 1 in, 3 out]
            n176 = call-poly "CSM - Filter JKISM String Queue.vi"("State(s) in (\"\")"=w400) -> ("States Out"=w399:string)  [unwired: 14 in]
            n177 = call "CSM - Forward UI Operations to CSM.vi"("Name(\"\" to use uuid)"=w397, "State(s) in (\"\")"=w399) -> ("States Out"=w398:string)  [unwired: 9 in]
          }
          event "Interface-Filter": Value Change {
            n178 = event-data() -> ()  [unwired: 1 in, 6 out]
            n179 = call <vilib>:"Add State(s) to Queue__JKI_lib_State_Machine.vi"("State(s) in Front (\"\")"="Action: Refresh Interface" ("State(s) in Front (\"\")"), "State(s) in (\"\")"=w403) -> ("States Out"=w404:string)  [unwired: 13 in]
          }
          event Panel Resize {
            # "Wait 50ms to prevent flood of events"
            n180 = event-data() -> ()  [unwired: 1 in, 3 out]
            n181 = call <vilib>:"Add State(s) to Queue__JKI_lib_State_Machine.vi"("State(s) in (\"\")"=w410, "State(s) at Back (\"\")"="//Panel Size Message to CSM" ("State(s) at Back (\"\")")) -> ("States Out"=w409:string)  [unwired: 13 in]
          }
          event Panel Close? {
            n182 = event-data() -> ()  [unwired: 1 in, 1 out]
            n183 = call "CSM - Forward UI Operations to CSM.vi"("Name(\"\" to use uuid)"=w413, "State(s) in (\"\")"="Macro: Exit" ("State")) -> ("States Out"=w412:string)  [unwired: 9 in]
            n184 = event-data("Discard?"=FALSE) -> ()  [unwired: 1 in, 1 out]
          }
          event "MainTree": Value Change {
            n185 = event-data() -> ()  [unwired: 1 in, 1 out]
            n186 = call "CSM - Convert Data to HexStr.vi"("Variant"="MainTree") -> ("HEX String (0-9,A-F)"=w417:string)  [unwired: 8 in]
            n187 = call <vilib>:"Build State String with Arguments__JKI_lib_State_Machine.vi"("Arguments (\"\")"=w417, "State"="Action: Refresh Interface") -> ("State with Arguments"=w419:string)  [unwired: 4 in]
            n188 = call <vilib>:"Add State(s) to Queue__JKI_lib_State_Machine.vi"("State(s) in Front (\"\")"=w419, "State(s) in (\"\")"=w421) -> ("States Out"=w422:string)  [unwired: 13 in]
          }
          event "MainTree": Shortcut Menu Activation? {
            n189 = event-data() -> ("CtlRef"=w424:refnum<vi>, "MenuRef"=w426:refnum<k9>, "Coords"=w425:T7)  [unwired: 1 in]
            n190 = call "_interfacebrowser Build MainTree Menu.vi"("CtlRef"=w424, "Coords"=w425, "Menu in"=w426) -> ("Discard?"=w427:bool)  [unwired: 8 in]
            n191 = event-data("Discard?"=w427) -> ()  [unwired: 1 in, 1 out]
          }
          event "CSM-States": Shortcut Menu Activation? {
            n192 = event-data() -> ("CtlRef"=w433:refnum<vi>, "MenuRef"=w434:refnum<k9>, "Coords"=w431:T7)  [unwired: 1 in, 4 out]
            n193 = control-ref of="MainTree"() -> (w430:refnum<vi>)
            n194 = call "_interfacebrowser Build Interface Menu.vi"("Tree"=w430, "CtlRef"=w433, "Coords"=w431, "Menu in"=w434) -> ("Discard?"=w432:bool)  [unwired: 7 in]
            n195 = event-data("Discard?"=w432) -> ()  [unwired: 1 in, 1 out]
          }
          event "MainTree": Shortcut Menu Selection (User) {
            n196 = event-data() -> ("ItemTag"=w438:string)  [unwired: 1 in, 7 out]
            n197 = call <vilib>:"Add State(s) to Queue__JKI_lib_State_Machine.vi"("State(s) in Front (\"\")"=w438, "State(s) in (\"\")"=w439, "State(s) at Back (\"\")"="Macro: Refresh UI" ("State(s) at Back (\"\")")) -> ("States Out"=w440:string)  [unwired: 12 in]
          }
          event "CSM-States": Shortcut Menu Selection (User) {
            n198 = event-data() -> ("ItemTag"=w444:string)  [unwired: 1 in, 7 out]
            n199 = Match Pattern(string=w444, regular expression="#") -> (before substring=w442:string)  [unwired: 1 in, 3 out]
            n200 = call <vilib>:"Add State(s) to Queue__JKI_lib_State_Machine.vi"("State(s) in Front (\"\")"=w442, "State(s) in (\"\")"=w446, "State(s) at Back (\"\")"="" ("State(s) at Back (\"\")")) -> ("States Out"=w447:string)  [unwired: 12 in]
          }
          event "MainTree": Mouse Move {
            n201 = event-data() -> ("CtlRef"=w455:refnum<vi>, "Coords"=w454:T7)  [unwired: 1 in, 3 out]
            n202 = invoke class="Tree (strict)" method="Point To Row Column"(reference=w455, "Point"=w454) -> ("Tag"=w452:string)  [unwired: 6 in, 7 out]
            n203 = Match Pattern(string=w452, regular expression="/") -> (before substring=w450:string)  [unwired: 1 in, 3 out]
            n204 = feedback-in #1(w450) -> ()
            n205 = feedback #1() -> (w451:string)  [unwired: 1 in]
            n206 = Not Equal?(x=w450, y=w451) -> (x != y?=w449:bool)
            n207 = case shown="True" w449 {
              tunnel: w450 -> [_ w459]
              frame False {
              }
              frame True {
                n208 = call "Read CSM-VI Info.vi"("CSM Name"=w459) -> ("Cluster 2"=w465:cluster{"Path":path})  [unwired: 9 in, 1 out]
                n209 = Unbundle By Name(w465) -> ("Path"=w464:path)
                n210 = Path To String(path=w464) -> (string=w463:string)
                n211 = call "lvcsm String to Path.vi"("common path"=w463) -> ("Path"=w462:path)  [unwired: 10 in]
                n212 = Path To String(path=w462) -> (string=w461:string)
                n213 = Concatenate Strings(w459, "  ----  " ("string"), w461) -> (→"String":string)
              }
            }
          }
          event "Refresh", "Opton:All-CSM-VIs": Value Change {
            n214 = event-data() -> ()  [unwired: 1 in, 1 out]
            n215 = call <vilib>:"Add State(s) to Queue__JKI_lib_State_Machine.vi"("State(s) in Front (\"\")"="Macro: Refresh UI" ("Init State(\"Macro: Initialize\")"), "State(s) in (\"\")"=w467) -> ("States Out"=w468:string)  [unwired: 13 in]
          }
          event "CSM-States": Double Click {
            n216 = event-data() -> ()  [unwired: 1 in, 5 out]
            n217 = call <vilib>:"Add State(s) to Queue__JKI_lib_State_Machine.vi"("State(s) in Front (\"\")"="Action: Refresh Image" ("State(s) in Front (\"\")"), "State(s) in (\"\")"=w471) -> ("States Out"=w472:string)  [unwired: 13 in]
          }
          event "Open": Value Change {
            n218 = event-data() -> ()  [unwired: 1 in, 1 out]
            n219 = call <vilib>:"Add State(s) to Queue__JKI_lib_State_Machine.vi"("State(s) in Front (\"\")"="ADD_CSMVI_ON_MAINTREEE" ("Init State(\"Macro: Initialize\")"), "State(s) in (\"\")"=w475) -> ("States Out"=w476:string)  [unwired: 13 in]
          }
          event "Scan Project": Value Change {
            n220 = event-data() -> ()  [unwired: 1 in, 5 out]
            n221 = call <vilib>:"Add State(s) to Queue__JKI_lib_State_Machine.vi"("State(s) in Front (\"\")"="SCAN_ALL_CSMVI\nMacro: Refresh UI" ("State(s) in Front (\"\")"), "State(s) in (\"\")"=w479) -> ("States Out"=w480:string)  [unwired: 13 in]
          }
          event User Event {
            n222 = event-data() -> ()  [unwired: 1 in, 1 out]
          }
        }
      }
      frame "Exit" {
        n223 = Unregister For Events(event registration refnum=w487) -> (error out=w486:errorcluster)  [unwired: 1 in]
        n224 = call <vilib>:"Clear Errors.vi"("error in (no error)"=w486) -> ()  [unwired: 5 in, 2 out]
      }
    }
  }
